vi "StartMeas.vi"(8 "error in (no error)":errorcluster, 10 "Variant":variant, 11 "NHRDCPower in":refnum<class "NHRDCPower.lvclass">) -> (0 "error out":errorcluster, 3 "NHRDCPower out":refnum<class "NHRDCPower.lvclass">)   [LabVIEW 2018, in "AcPwrPlugins.lvlib" / "NHRDCPower.lvclass"]
doc: "This VI initiates the measurement on the instrument(s)."
uses:
  NHRDCPower.lvclass
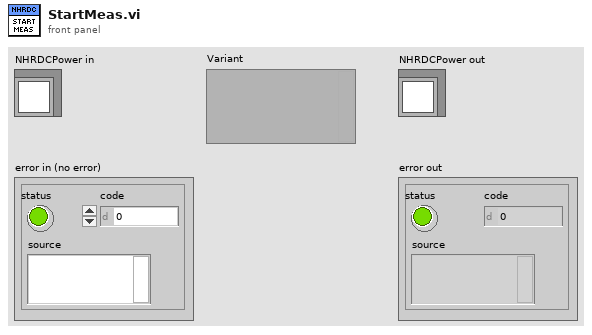
[diagram p1: front panel]
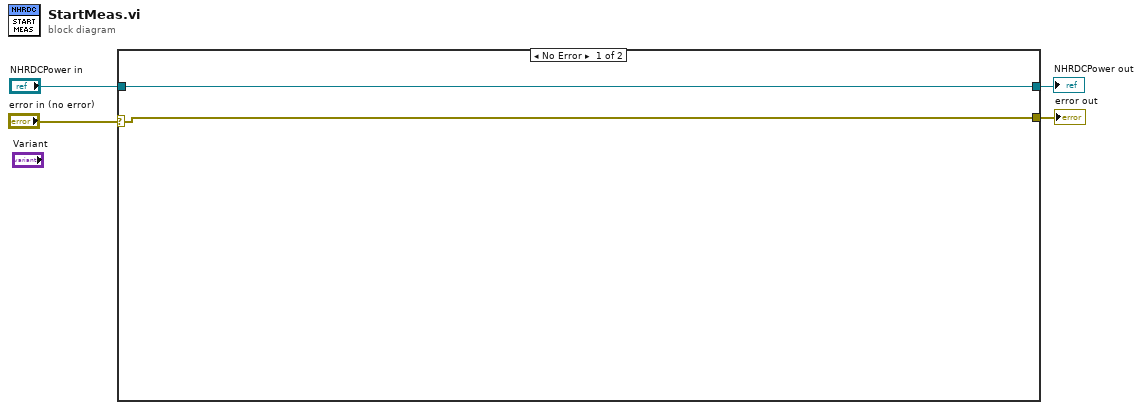
[diagram p0: block diagram]
diagram:
  n1 = case shown="No Error" "error in (no error)" {
    selector: "error in (no error)" -> [w5 w7]
    tunnel: [w5 w7] -> w3
    tunnel: [w6 w8] -> w4
    tunnel: "NHRDCPower in" -> [w6 w8]
    frame No Error {
    }
    frame Error {
    }
  }
  "error out" <- w3
  "NHRDCPower out" <- w4
